vi "Dimmer_PS.vi"   [LabVIEW 2012]
types:
  T1 = typedef "BotSpeak_Control.ctl" = cluster{"Address":string, "Reply EOF":string, "Hardware":string, "Retries":i8, "Timeout":i32}
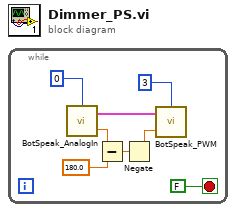
[diagram p0: block diagram]
diagram:
  n1 = while {
    stop <- FALSE stop-if-true
    n2 = call <userlib>:"BotSpeak_AnalogIn.vi"("A/D Channel"=u8 0) -> ("voltage"=w5:dbl, "Bot Settings"=w6:T1)  [unwired: 2 in]
    n3 = Subtract(x=w5, y=180.0) -> (x-y=w3:dbl)
    n4 = Negate(x=w3) -> (-x=w2:dbl)
    n5 = call <userlib>:"BotSpeak_PWM.vi"("Strength (100)"=w2, "Bot Settings"=w6, "PWM Line"=u8 3 ("DAC Channel")) -> ()  [unwired: 2 out]
  }
